vi "isTerminate.vi"(0 "object in":refnum<class "NewOff1.lvclass">, 5 "error in (no error)":errorcluster) -> (14 "object out":refnum<class "NewOff1.lvclass">, 19 "error out":errorcluster)   [LabVIEW 2022 SP3, in "NewOff1.lvclass"]
uses:
  NewOff1.lvclass
  Play_class/Play.lvclass
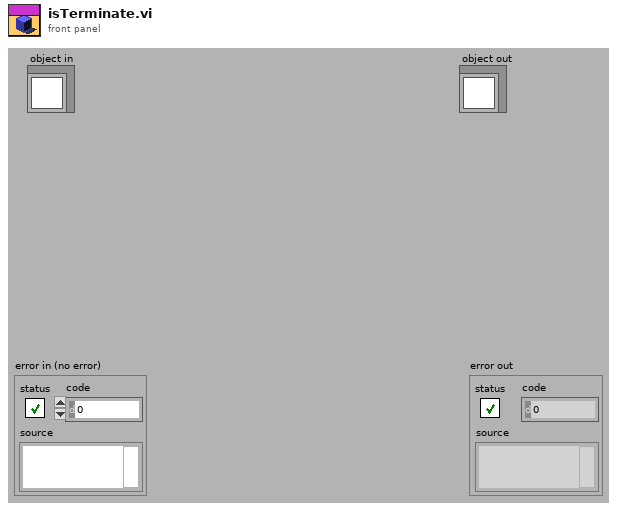
[diagram p1: front panel]
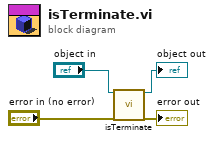
[diagram p0: block diagram]
diagram:
  n1 = call-parent "isTerminate.vi"("object in"="object in", "error in (no error)"="error in (no error)") -> ("object out"=→"object out":refnum<class "NewOff1.lvclass">, "error out"=→"error out":errorcluster)  [unwired: 16 in]
